vi "load setpoint code.vi"(6 "Load or config":enum16{"load", "configure"}(ring), 8 "index":i32, 9 "Set Points":T2[](array[typedef]) {"value" format="%#_6p"; "variable"."Data average interval" min=0.0 format="%^#_3g"}) -> (0 "setpoint match":T1, 1 "Set Points out":T2[](array[typedef]) {"value" format="%#_6p"; "variable"."Data average interval" min=0.0 format="%^#_3g"})   [LabVIEW 2012]
uses:
  type specifier for control code.ctl
  variable setpoint.ctl
  data ave interval.ctl
  setpoint match.ctl
panel:
  in  "type specifier VI Refnum (for type only)":T4
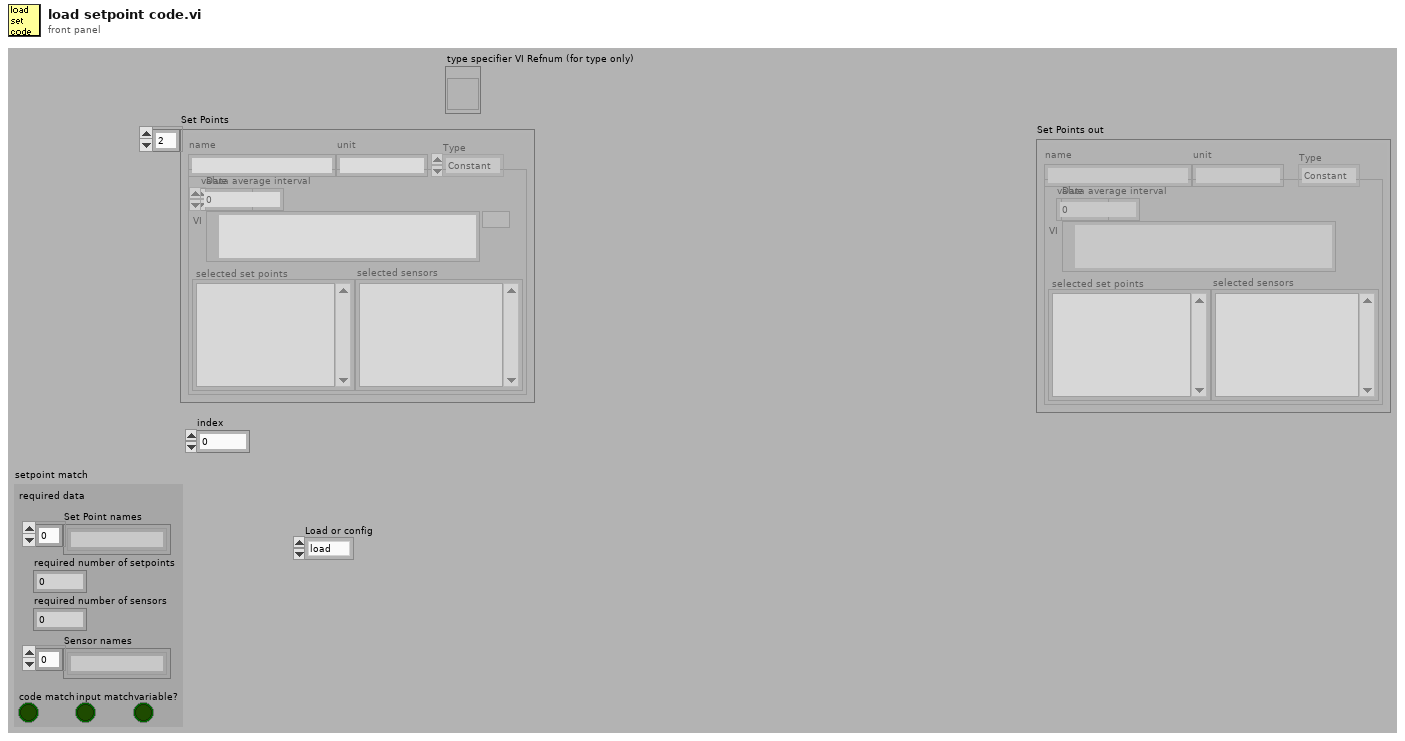
[diagram p1: front panel]
types:
  T1 = typedef "setpoint match.ctl" = cluster{"required data":cluster{"Set Point names":string[], "required number of setpoints":u8, "required number of sensors":u8, "Sensor names":string[]}, "input match":bool, "code match":bool, "variable?":bool}
  T2 = typedef "variable setpoint.ctl" = cluster{"name":string, "unit":string, "value":dbl, "Type":enum16{"Constant", "Variable"}, "variable":cluster{"selected sensors":i32[], "selected set points":i32[], "VI":path, "Data average interval":T3, "code ref":T4}}
  T3 = typedef "data ave interval.ctl" = dbl
  T4 = typedef "type specifier for control code.ctl" = refnum<vi>
  T5 = cluster{"Set Point names":string[], "required number of setpoints":u8, "required number of sensors":u8, "Sensor names":string[]}
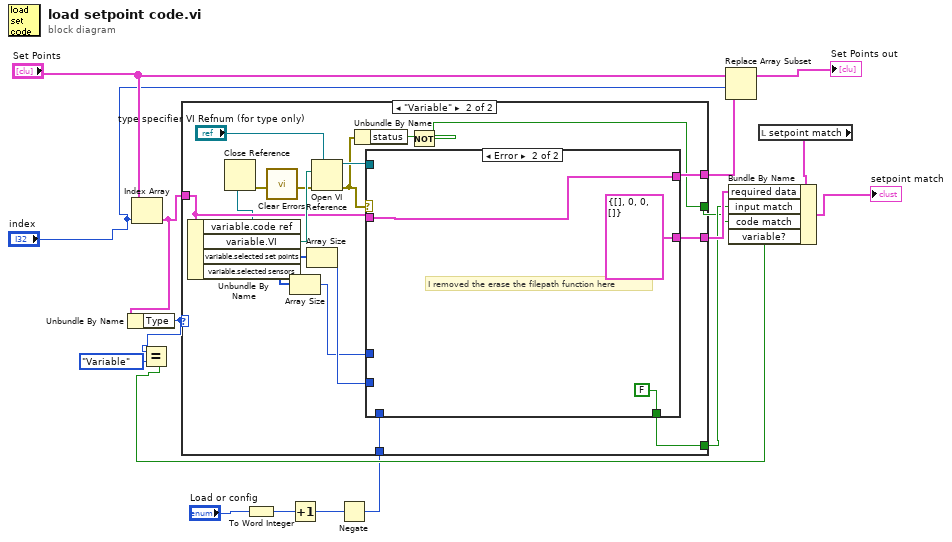
[diagram p0: block diagram]
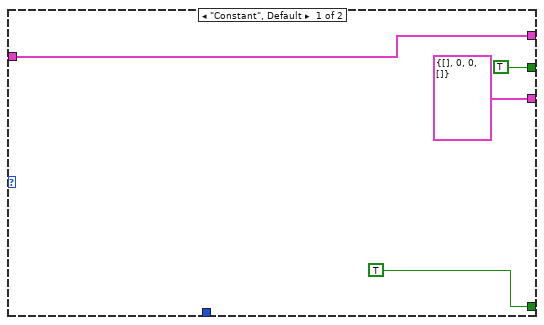
[diagram p2: hidden frame]
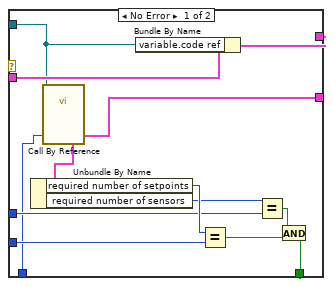
[diagram p3: hidden frame]
diagram:
  n1 = Index Array(array="Set Points", index="index") -> (element=w17:T2)
  n2 = Unbundle By Name(w17) -> ("Type"=w12:enum16{"Constant", "Variable"})
  n3 = Equal?(x=w12, y=enum16{"Constant", "Variable"}."Variable") -> (x = y?=w5:bool)
  n4 = To Word Integer(number="Load or config") -> (16bit integer=w2:i16)
  n5 = Increment(x=w2) -> (x+1=w3:i16)
  n6 = Negate(x=w3) -> (-x=w1:i16)
  n7 = case shown="\"Variable\"" w12 {
    tunnel: w17 -> [w21 w38]
    tunnel: [w21 w36] -> w13
    tunnel: [TRUE w35] -> w7
    tunnel: [T5 {"Set Point names"=[], "required number of setpoints"=0, "required number of sensors"=0, "Sensor names"=[]} ("required data") w24] -> w8
    tunnel: [TRUE w23] -> w6
    tunnel: w1 -> [_ w22]
    frame "Constant", Default {
    }
    frame "Variable" {
      n8 = Unbundle By Name(w38) -> ("variable.code ref"=w27:T4, "variable.VI"=w39:path, "variable.selected set points"=w33:i32[], "variable.selected sensors"=w31:i32[])
      n9 = Close Reference(reference=w27) -> (error out=w26:errorcluster)  [unwired: 1 in]
      n10 = call <vilib>:"Clear Errors.vi"("error in (no error)"=w26) -> ("error out"=w25:errorcluster)  [unwired: 6 in]
      n11 = Array Size(array=w31) -> (size(s)=w30:i32)
      n12 = Array Size(array=w33) -> (size(s)=w32:i32)
      n13 = Open VI Reference(type specifier VI Refnum (for type only)="type specifier VI Refnum (for type only)", vi path=w39, error in (no error)=w25) -> (vi reference=w37:T4, error out=w29:errorcluster)  [unwired: 3 in]
      n14 = Unbundle By Name(w29) -> ("status"=w28:bool)
      n15 = case shown="Error" w29 {
        tunnel: w38 -> [w51 w52]
        tunnel: w37 -> [w49 _]
        tunnel: [w50 w52] -> w36
        tunnel: [w43 FALSE] -> w35
        tunnel: w32 -> [w48 _]
        tunnel: w30 -> [w42 _]
        tunnel: [w41 T5 {"Set Point names"=[], "required number of setpoints"=0, "required number of sensors"=0, "Sensor names"=[]} ("required data")] -> w24
        tunnel: w22 -> [w40 _]
        frame No Error {
          n16 = call-by-ref "?"(reference=w49, "State"=w40) -> ("required data"=w41:T5)  [unwired: 6 in, 3 out]
          n17 = Unbundle By Name(w41) -> ("required number of setpoints"=w47:u8, "required number of sensors"=w46:u8)
          n18 = Bundle By Name(cluster=w51, "variable.code ref"=w49) -> (w50:T2)
          n19 = Equal?(x=w47, y=w48) -> (x = y?=w44:bool)
          n20 = Equal?(x=w46, y=w42) -> (x = y?=w45:bool)
          n21 = And(x=w45, y=w44) -> (x .and. y?=w43:bool)
        }
        frame Error {
          # "I removed the erase the filepath function here"
        }
      }
      n22 = Not(x=w28) -> (.not. x?=w23:bool)
    }
  }
  n23 = Replace Array Subset(array="Set Points", new element=w13, index="index") -> (→"Set Points out":T2[])
  n24 = local read "setpoint match"() -> (w10:T1)
  n25 = Bundle By Name(cluster=w10, "required data"=w8, "input match"=w7, "code match"=w6, "variable?"=w5) -> (→"setpoint match":T1)
